vi "SetIntegrationTime.vi"(8 "error in":errorcluster, 10 "ExposureTime(mSec)":dbl, 11 "VISAresource":refnum<visa-resource-name>) -> (0 "error out":errorcluster, 3 "ExposureTimeReadout(mSec)":dbl)   [LabVIEW 2020]
doc: "Send and read-back the exposure time to/from the device connected to the specified VISAresource"
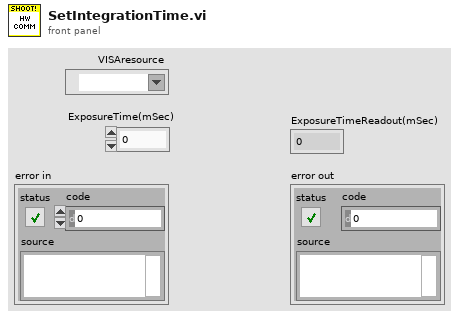
[diagram p1: front panel]
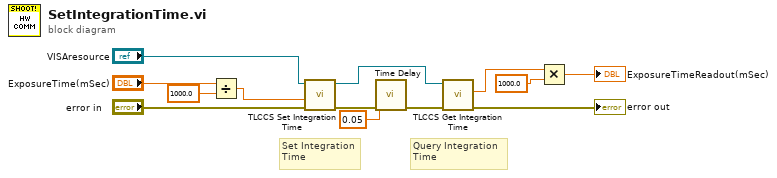
[diagram p0: block diagram]
diagram:
  # "Query Integration\nTime"
  # "Set Integration\nTime"
  n1 = Divide(x="ExposureTime(mSec)", y=1000.0) -> (x/y=w3:dbl)
  n2 = call "TLCCS Set Integration Time.vi"("error in (no error)"="error in", "Integration Time [s] (0.001)"=w3, "instrument handle"="VISAresource") -> ("error out"=w5:errorcluster, "instrument handle out"=w7:refnum<visa-resource-name>)  [unwired: 7 in]
  n3 = call "Time Delay"("error in (no error)"=w5, "Delay Time (s)"=0.05) -> ("error out"=w6:errorcluster)  [unwired: 9 in]
  n4 = call "TLCCS Get Integration Time.vi"("error in (no error)"=w6, "instrument handle"=w7) -> ("error out"=→"error out":errorcluster, "Integration Time [s]"=w10:dbl)  [unwired: 7 in, 1 out]
  n5 = Multiply(x=w10, y=1000.0) -> (x*y=→"ExposureTimeReadout(mSec)":dbl)
